vi "stopXY_img.vi"   [LabVIEW 2013]
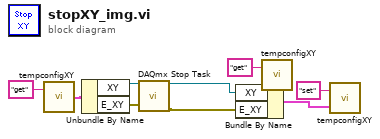
[diagram p0: block diagram]
diagram:
  n1 = call "tempconfigXY.vi"("command"="get") -> ("Temp Config out"=w4:cluster{" XY":refnum<k21>, "E_XY":errorcluster})  [unwired: 1 in]
  n2 = Unbundle By Name(w4) -> ("XY"=w5:refnum<k21>, "E_XY"=w6:errorcluster)
  n3 = call <vilib>:"DAQmx Stop Task.vi"("task/channels in"=w5, "error in"=w6) -> ("task out"=w1:refnum<k21>, "error out"=w2:errorcluster)  [unwired: 12 in]
  n4 = call "tempconfigXY.vi"("command"="get") -> ("Temp Config out"=w9:cluster{" XY":refnum<k21>, "E_XY":errorcluster})  [unwired: 1 in]
  n5 = Bundle By Name(cluster=w9, "XY"=w1, "E_XY"=w2) -> (w10:cluster{" XY":refnum<k21>, "E_XY":errorcluster})
  n6 = call "tempconfigXY.vi"("Temp Config in"=w10, "command"="set") -> ()  [unwired: 1 out]
